vi "P1_1_ModosAccion.vi"() -> ()   [LabVIEW 2020]
panel:
  out "Respuesta \nString":string
  in  "String":string
  out "Respuesta\nBoolean":bool
  in  "Boolean":bool
  out "Respuesta \nSlide":dbl
  out "Respuesta \nScrollbar":dbl
  out "Respuesta \nDial":dbl
  out "Respuesta\nNumeric":dbl
  in  "Scrollbar":i32(c297)
  in  "Slide":dbl(slide) scale=0.0..10.0
  in  "Dial":dbl(knob) scale=0.0..10.0
  in  "Numeric":dbl
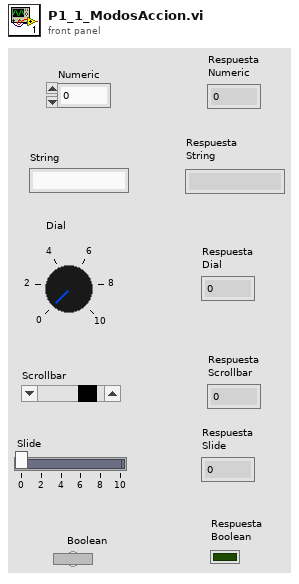
[diagram p1: front panel]
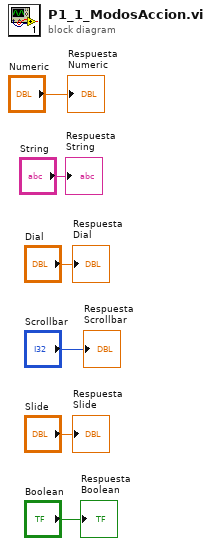
[diagram p0: block diagram]
diagram:
  "Respuesta\nNumeric" <- "Numeric"
  "Respuesta \nDial" <- "Dial"
  "Respuesta \nScrollbar" <- "Scrollbar"
  "Respuesta \nSlide" <- "Slide"
  "Respuesta\nBoolean" <- "Boolean"
  "Respuesta \nString" <- "String"
